vi "Simple UDP - Receiver.vi"() -> ()   [LabVIEW 2018]
doc: "The UDP protocol differs from TCP in that there is no error-checking with the packets of information that are sent, and thus no guarantee whatsoever that an intended recipient will actually receive a given piece of data.\n\nUDP does offer the ability to \"broadcast\" data across a network--simply specify an IP Address of all ones (255.255.255.255) to attempt to broadcast information network-wide. Keep in mind that routers and other network hardware will generally refuse to forward the broadcast beyond certain points, so the extent of the broadcast will in practice be limited."
panel:
  out "Anzahl":i32
  out "Verpasst?":u32
  out "Zeitdifferenz [msec]":dbl format="%.2f"
  out "Gauge":i32(knob) scale=0.0..60.0
  out "Received Data":i32(graph)
  in  "Stop":bool
  # "Überblick Simple UDP - Receiver.vi  zeigt UDP - Kommunikation. Das ist hier der Empfänger. Das Zeitdifferenz zwischen zwei Messages wird angezeigt. \nAnleitung:\nSimple UDP - Sender.vi läuft schon oder wird später gestartet und sendet eine Zahl pro Sekunde.\nDownload dieses VI auf das myRIO(SUNderbird1)"
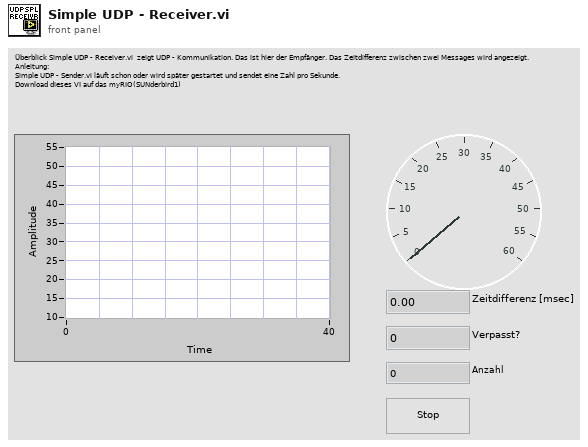
[diagram p1: front panel]
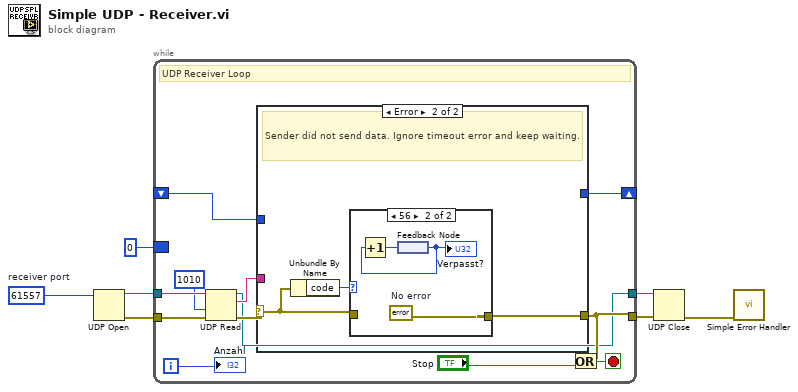
[diagram p0: block diagram]
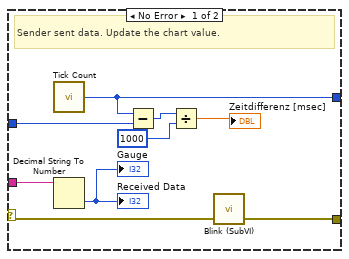
[diagram p2: hidden frame]
diagram:
  w3 = u16 61557  # receiver port
  n1 = UDP Open(11:w3) -> (port=w4:refnum<k16>, 0:w5:errorcluster)  [unwired: 4 in, 1 out]
  n2 = while {
    tunnel: w4 -> [w19]
    tunnel: [w11] -> w7
    tunnel: w5 -> [w16]
    tunnel: [w12] -> w6
    shift-right: [w9] -> _
    shift-left: _ -> [w10]
    border: u32 0 -> [_]
    i -> [w8]
    stop <- w17 stop-if-true
    # "UDP Receiver Loop"
    n3 = UDP Read(connection ID=w19, timeout ms (25000)=1010, 8:w16) -> (data out=w14:string, error out=w13:errorcluster, 3:w11:refnum<k16>)  [unwired: 3 out]
    n4 = case shown="Error" w13 {
      selector: w13 -> [w22 w29]
      tunnel: w14 -> [w27 _]
      tunnel: [w23 w30] -> w12
      tunnel: w10 -> [w26 _]
      tunnel: [w25 _] -> w9
      frame No Error {
        # "Sender sent data. Update the chart value."
        n5 = call "Tick Count"() -> ("Tick Count(uSec)"=w25:u32)
        n6 = Decimal String To Number(string=w27) -> (number=→"Received Data" →"Gauge":i32)  [unwired: 2 in, 1 out]
        n7 = Subtract(x=w25, y=w26) -> (x-y=w24:u32)
        n8 = Divide(x=w24, y=u32 1000) -> (x/y=→"Zeitdifferenz [msec]":dbl)
        n9 = call "Blink (SubVI).vi"("error in (no error)"=w22) -> ("error out"=w23:errorcluster)  [unwired: 2 in]
      }
      frame Error {
        # "Sender did not send data. Ignore timeout error and keep waiting."
        n10 = Unbundle By Name(w29) -> ("code"=w31:i32)
        n11 = case shown="56" w31 {
          tunnel: w29 -> [w32 _]
          tunnel: [w32 w35] -> w30
          frame Default {
          }
          frame 56 {
            w35 = errorcluster {"status"=FALSE, "code"=0, "source"=""}  # No error
            n12 = feedback #1() -> (w33:u32)
            "Verpasst?" <- w33
            n13 = Increment(x=w33) -> (x+1=w34:u32)
            n14 = feedback-in #1(w34) -> ()
          }
        }
      }
    }
    n15 = Or(x=w12, y="Stop") -> (x .or. y?=w17:bool)
    "Anzahl" <- w8
  }
  n16 = UDP Close(connection ID=w7, 8:w6) -> (error out=w2:errorcluster)  [unwired: 1 out]
  n17 = call <vilib>:"Simple Error Handler.vi"("error in (no error)"=w2) -> ()  [unwired: 1 in, 8 out]
